vi "Query Next Example.vi"() -> ()   [LabVIEW 2020, in "ORM_Examples.lvlib"]
doc: "Returns the first two row results from the result set of the query using the \"Next\" function. Note that bbPlayers and BB Players Map are not needed for this example."
uses:
  ORM_Examples.lvlib
  <vilib>/Viviota/shared/ORM.lvlibp/ORM/TypeMap/TypeMap.lvclass
  e0c6de7d-38cb-4ce3-8c6b-1f4449f31f0b.vi
  e0c6de7d-38cb-4ce3-8c6b-1f4449f31f0b.vi/898c9d12-c4a1-4fc2-b53a-10a82e67b237.vi
  e0c6de7d-38cb-4ce3-8c6b-1f4449f31f0b.vi/b8e1d063-fe91-4644-90c0-977cc91ec382.vi
  <vilib>/Viviota/shared/ORM_ADONet.lvlibp/ADOMapper/ADOMapper.lvclass
  C:/Program Files/National Instruments/LabVIEW 2024/vi.lib/Viviota/shared/ORM.lvlibp/ORM/SqlMapper/SqlMapper.lvclass
  <vilib>/Viviota/shared/ORM.lvlibp/ORM/TypeMap/Write Table Name.vi
  <vilib>/Viviota/shared/ORM_DBC_Sqlite.lvlibp/Sqlite Connect.vi
  <vilib>/Utility/error.llb/Error Cluster From Error Code.vi
  <vilib>/Viviota/shared/ORM.lvlibp/ORM/TypeMap/Read TypeMap.vi
  <vilib>/Viviota/shared/ORM.lvlibp/ORM/TypeMap/ToLabVIEW_Wrap.vi
  <vilib>/Viviota/shared/ORM.lvlibp/ORM/Query Result/Query Result.lvclass
  ORM_API/ORM_API.lvlib
  <vilib>/Viviota/shared/ORM_ADONet.lvlibp
  <vilib>/Viviota/shared/ORM_DBC_Sqlite.lvlibp/DBC.lvclass
  <vilib>/Viviota/shared/ORM.lvlibp/ORM/DynamicParameters/DynamicParameters.lvclass
  C:/Program Files/National Instruments/LabVIEW 2024/vi.lib/Viviota/shared/ORM_ADONet.lvlibp/ADOMapper/ADOMapper.lvclass
panel:
  out "foundSecond?":bool=TRUE
  out "Second Row":variant
  out "foundFirst?":bool=TRUE
  out "First Row":variant
  in  "SQL Query":string
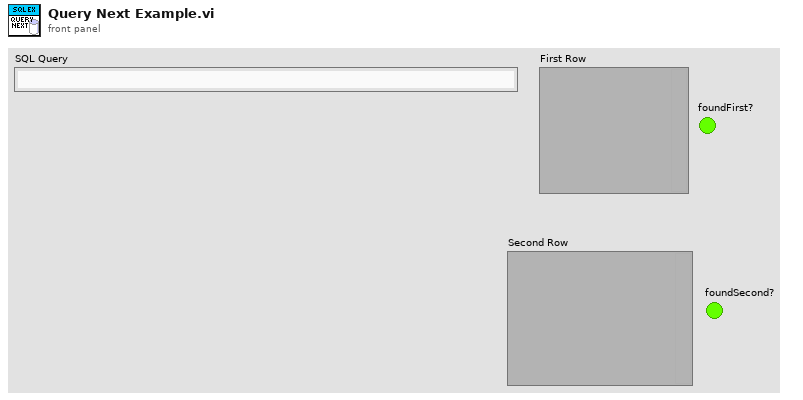
[diagram p1: front panel]
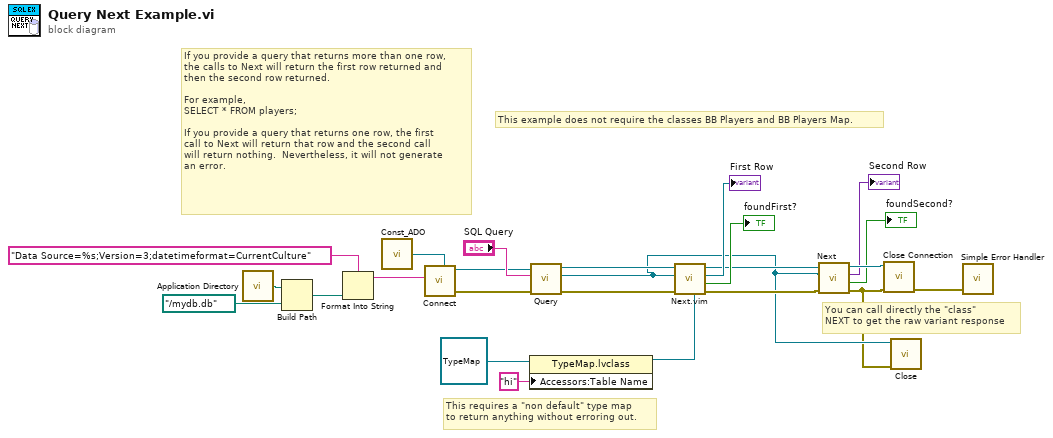
[diagram p0: block diagram]
diagram:
  # "You can call directly the \"class\" \nNEXT to get the raw variant response"
  # "This requires a \"non default\" type map\nto return anything without erroring out."
  # "This example does not require the classes BB Players and BB Players Map."
  # "If you provide a query that returns more than one row,\nthe calls to Next will return the first row returned and\nthen the second row returned.\n\nFor example,\nSELECT * FROM players;\n\nIf you provide a query that returns one row, the first \ncall to Next will return that row and the second call\nwill return nothing.  Nevertheless, it will not generate\nan error."
  n1 = call <vilib>:"Application Directory.vi"() -> ("Application Directory"=w15:path)
  n2 = Build Path(base path=w15, name or relative path=path "../mydb.db" ("file out")) -> (appended path=w16:path)
  n3 = Format Into String(format string="Data Source=%s;Version=3;datetimeformat=CurrentCulture" ("connectionStringName"), w16) -> (resulting string=w11:string)  [unwired: 2 in, 1 out]
  n4 = call <vilib>:"Const_ADO.vi"() -> ("ADOMapper"=w12:refnum<class "ADOMapper.lvclass">)
  n5 = call-poly "Connect.vi"("SqlMapper Type"=w12, "Connection String"=w11) -> ("error out"=w9:errorcluster, "SqlMapper out"=w10:refnum<class "ADOMapper.lvclass">)  [unwired: 8 in]
  n6 = property class="TypeMap.lvclass"(reference=refnum<class "TypeMap.lvclass"> refnum ("Dapper.lvlib:TypeMap.lvclass"), "Accessors:Table Name"="hi" ("Table Name")) -> (reference out=w19:refnum<class "TypeMap.lvclass">)  [unwired: 1 in, 1 out]
  n7 = call-dynamic "Query.vi"("error in (no error)"=w9, "sql"="SQL Query", "ADOMapper in"=w10) -> ("error out"=w24:errorcluster, "Query Result out"=w2:refnum<class "Query Result.lvclass">, "ADOMapper out"=w22:refnum<class "ADOMapper.lvclass">)  [unwired: 6 in]
  n8 = call "Next.vim"("TypeMap in"=w19, "error in (no error)"=w24, "Query in"=w2, "SqlMapper in"=w22) -> ("error out"=w3:errorcluster, "found?"=→"foundFirst?":bool, "Row"=→"First Row":refnum<class>, "SqlMapper out"=w8:refnum<class "SqlMapper.lvclass">)  [unwired: 4 in]
  n9 = call <vilib>:"Next.vi"("error in (no error)"=w3, "Query in"=w2, "SqlMapper in"=w8) -> ("error out"=w1:errorcluster, "found?"=→"foundSecond?":bool, "Row"=→"Second Row":variant, "SqlMapper out"=w7:refnum<class "SqlMapper.lvclass">)  [unwired: 5 in]
  n10 = call "Close Connection.vi"("Error In"=w1, "SqlMapper"=w7) -> ("Error Out"=w5:errorcluster)  [unwired: 9 in]
  n11 = call-dynamic "Close.vi"("error in (no error)"=w1, "Query Result in"=w2) -> ()  [unwired: 9 in, 1 out]
  n12 = call <vilib>:"Simple Error Handler.vi"("error in (no error)"=w5) -> ()  [unwired: 4 in, 5 out]
